vi "GetPolygonPointsBetweenSides.vi"(1 "Polygon":T2, 2 "LastSideIndex":i32, 3 "FirstSideIndex":i32) -> (0 "PolygonVertices":T1[](array[typedef]))   [LabVIEW 2017, in "ArgosLib.lvlib"]
uses:
  ArgosLib.lvlib
  TypeDefs/Polygon2D.ctl
  TypeDefs/Point2D.ctl
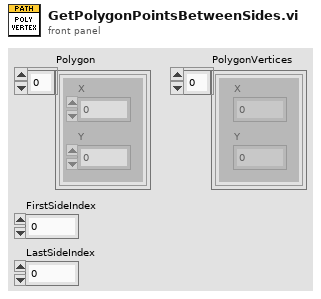
[diagram p1: front panel]
types:
  T1 = typedef "ArgosLib.lvlib/Point2D.ctl" = cluster{"X":dbl, "Y":dbl}
  T2 = typedef "ArgosLib.lvlib/Polygon2D.ctl" = T1[]
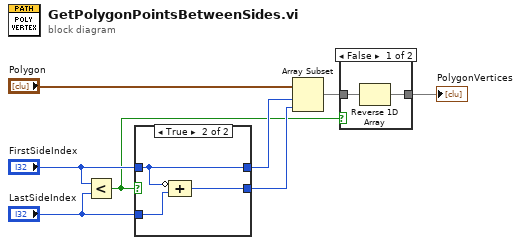
[diagram p0: block diagram]
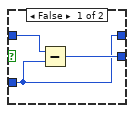
[diagram p3: hidden frame]
diagram:
  n1 = Less?(x="FirstSideIndex", y="LastSideIndex") -> (x < y?=w1:bool)
  n2 = case shown="True" w1 {
    tunnel: "FirstSideIndex" -> [w11 w12]
    tunnel: "LastSideIndex" -> [w9 w14]
    tunnel: [w10 w13] -> w5
    tunnel: [w9 w12] -> w4
    frame False {
      n3 = Subtract(x=w11, y=w9) -> (x-y=w10:i32)
    }
    frame True {
      n4 = Compound Arithmetic op=ADD(invert w12, w14) -> (w13:i32)
    }
  }
  n5 = Array Subset(array="Polygon", index=w4, length=w5) -> (w3:T2)
  n6 = case shown="False" w1 {
    tunnel: [w15 w17] -> w2
    tunnel: w3 -> [w16 w17]
    frame False {
      n7 = Reverse 1D Array(array=w16) -> (reversed array=w15:T2)
    }
    frame True {
    }
  }
  "PolygonVertices" <- w2
